vi "laser_test.vi"() -> ()   [LabVIEW 2011]
uses:
  <vilib>/Analysis/NI_AALBase.lvlib
panel:
  in  "stop":bool
  out "Photodiode Voltage":dbl(graph)
  out "Average Voltage Out":dbl format="%0.2f"
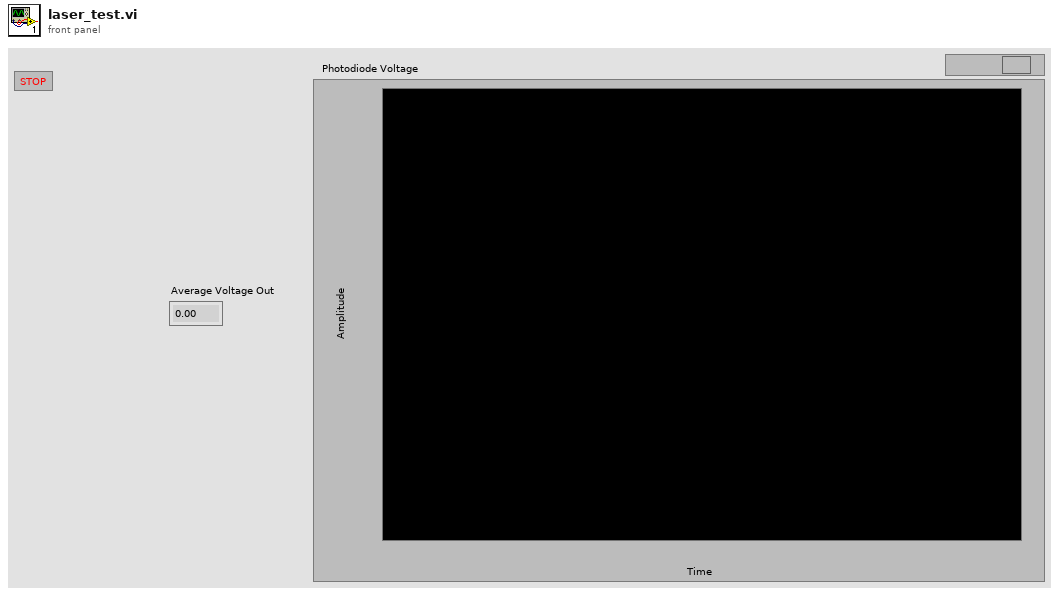
[diagram p1: front panel]
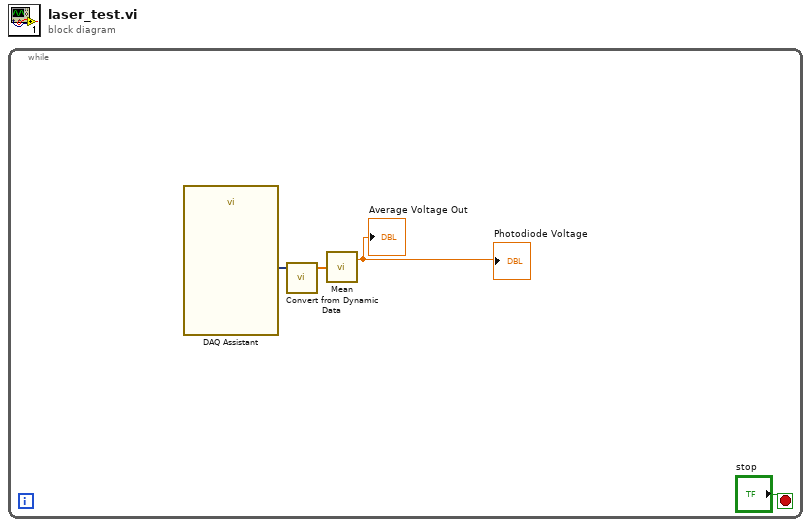
[diagram p0: block diagram]
diagram:
  n1 = while {
    stop <- "stop" stop-if-true
    n2 = call "DAQ Assistant"() -> ("data"=w3:dynamicdata)  [unwired: 17 in, 2 out]
    n3 = call "Convert from Dynamic Data"("Dynamic Data Type"=w3) -> ("Array"=w4:dbl[])  [unwired: 3 in]
    n4 = call <vilib>:"Mean.vi"("X"=w4) -> ("mean"=→"Average Voltage Out" →"Photodiode Voltage":dbl)  [unwired: 1 out]
  }
